vi "Service Request Handler.vi"(6 "Check address? (False)":bool, 8 "Error In (No Error)":errorcluster, 9 "Expected Sensor Address (a)":string="a", 10 "Service Request":string, 11 "RS232 Port In":refnum<visa-resource-name>) -> (0 "Error Out":errorcluster, 1 "Address Match?":bool, 2 "Sensor Address Out":string, 3 "RS232 Port Out":refnum<visa-resource-name>)   [LabVIEW 2016, in "SDI-12.lvlib"]
doc: "Handles sensor replies to service requests, which are generic messages for a variety SDI-12 commands.\n\nResponse format: a<CR><LF>\n\nWhere 'a' represents the sensor address.\n\nThe following commands result in a service request by the sensor:\n1. Acknowledge Active\n2. Change Address (with new address).\n3. Address Query.\n4. Normal Measurements (as opposed to concurrent or continuous. Additional Measurements could be either normal or concurrent).\n5. When a sensor is sent a command that it does not support."
uses:
  SDI-12.lvlib
panel:
  # "SDI-12 Service Request = a<CR><LF>\nWhere a = a valid SDI-12 address"
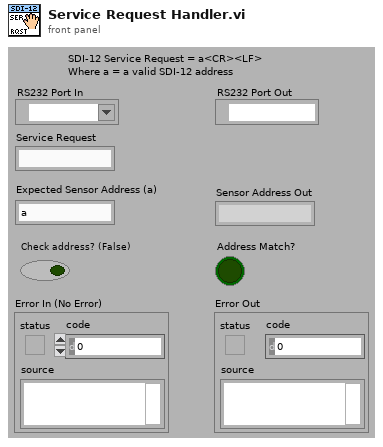
[diagram p1: front panel]
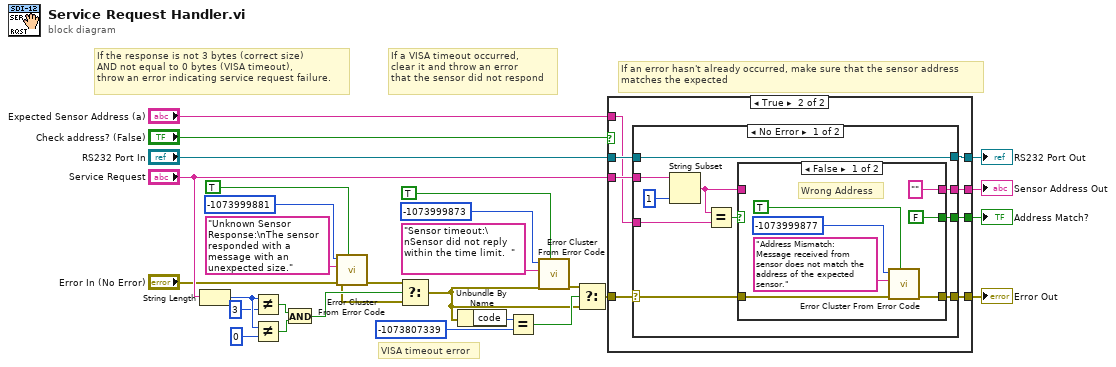
[diagram p0: block diagram]
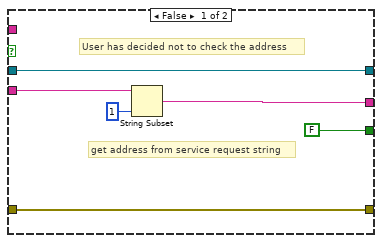
[diagram p2: hidden frame]
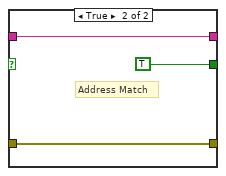
[diagram p3: hidden frame]
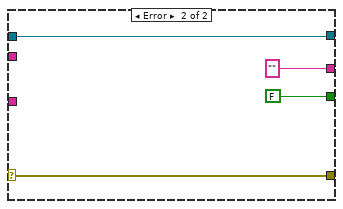
[diagram p4: hidden frame]
diagram:
  # "If an error hasn't already occurred, make sure that the sensor address\nmatches the expected"
  # "VISA timeout error"
  # "If a VISA timeout occurred, \nclear it and throw an error\nthat the sensor did not respond"
  # "If the response is not 3 bytes (correct size) \nAND not equal to 0 bytes (VISA timeout),\nthrow an error indicating service request failure."
  n1 = String Length(string="Service Request") -> (length=w23:i32)
  n2 = Not Equal?(x=w23, y=3) -> (x != y?=w25:bool)
  n3 = Not Equal?(x=w23, y=0) -> (x != y?=w26:bool)
  n4 = And(x=w25, y=w26) -> (x .and. y?=w4:bool)
  n5 = call <vilib>:"Error Cluster From Error Code.vi"("show call chain? (False)"=TRUE ("Error?"), "error in (no error)"="Error In (No Error)", "error message (\"\")"="Unknown Sensor Response:\nThe sensor responded with a message with an unexpected size." ("error message (\"\")"), "error code (0)"=-1073999881 ("error code")) -> ("error out"=w5:errorcluster)  [unwired: 5 in]
  n6 = Select(t=w5, s=w4, f="Error In (No Error)") -> (s? t:f=w3:errorcluster)
  n7 = Unbundle By Name(w3) -> ("code"=w28:i32)
  n8 = Equal?(x=w28, y=-1073807339) -> (x = y?=w8:bool)
  n9 = call <vilib>:"Error Cluster From Error Code.vi"("show call chain? (False)"=TRUE, "error in (no error)"=w3, "error message (\"\")"="Sensor timeout:\nSensor did not reply within the time limit.  " ("error message (\"\")"), "error code (0)"=-1073999873 ("error code")) -> ("error out"=w7:errorcluster)  [unwired: 5 in]
  n10 = Select(t=w7, s=w8, f=w3) -> (s? t:f=w6:errorcluster)
  n11 = case shown="True" "Check address? (False)" {
    tunnel: w6 -> [w33 w42]
    tunnel: "RS232 Port In" -> [w34 w41]
    tunnel: [w34 w40] -> w20
    tunnel: [w33 w39] -> w19
    tunnel: [w31 w38] -> w18
    tunnel: "Service Request" -> [w29 w37]
    tunnel: [FALSE w36] -> w15
    tunnel: "Expected Sensor Address (a)" -> [_ w35]
    frame False {
      # "get address from service request string"
      # "User has decided not to check the address"
      n12 = String Subset(string=w29, length (rest)=1 ("length (rest)")) -> (substring=w31:string)  [unwired: 1 in]
    }
    frame True {
      n13 = case shown="No Error" w42 {
        selector: w42 -> [w50 w66]
        tunnel: w41 -> [w51 w64]
        tunnel: [w51 w64] -> w40
        tunnel: [w49 w66] -> w39
        tunnel: [w48 "" ("sensor address out")] -> w38
        tunnel: w37 -> [w46 _]
        tunnel: [w44 FALSE] -> w36
        tunnel: w35 -> [w43 _]
        frame No Error {
          n14 = String Subset(string=w46, length (rest)=1 ("length (rest)")) -> (substring=w47:string)  [unwired: 1 in]
          n15 = Equal?(x=w47, y=w43) -> (x = y?=w45:bool)
          n16 = case shown="False" w45 {
            tunnel: [w57 w62] -> w49
            tunnel: w50 -> [w53 w62]
            tunnel: ["" ("sensor address out") w61] -> w48
            tunnel: w47 -> [_ w61]
            tunnel: [FALSE TRUE] -> w44
            frame False {
              # "Wrong Address"
              n17 = call <vilib>:"Error Cluster From Error Code.vi"("show call chain? (False)"=TRUE ("Error?"), "error in (no error)"=w53, "error message (\"\")"="Address Mismatch:  Message received from sensor does not match the address of the expected sensor." ("error message (\"\")"), "error code (0)"=-1073999877 ("error code")) -> ("error out"=w57:errorcluster)  [unwired: 5 in]
            }
            frame True {
              # "Address Match"
            }
          }
        }
        frame Error {
        }
      }
    }
  }
  "RS232 Port Out" <- w20
  "Error Out" <- w19
  "Sensor Address Out" <- w18
  "Address Match?" <- w15
